vi "set C1 trigger.vi"(8 "error in (no error)":errorcluster, 10 "free run?":bool, 11 "Waveform in":refnum<class "Waveform.lvclass">) -> (0 "error out":errorcluster, 3 "Waveform out":refnum<class "Waveform.lvclass">)   [LabVIEW 2012, in "Waveform.lvclass"]
uses:
  Waveform.lvclass
  Waveform.lvclass/Waveform.ctl
  <vilib>/DAQmx/configure/trigger.llb/DAQmx Start Trigger (Digital Edge).vi
  <vilib>/DAQmx/configure/trigger.llb/DAQmx Start Trigger (None).vi
  <resource>/objmgr/daqmx.rc
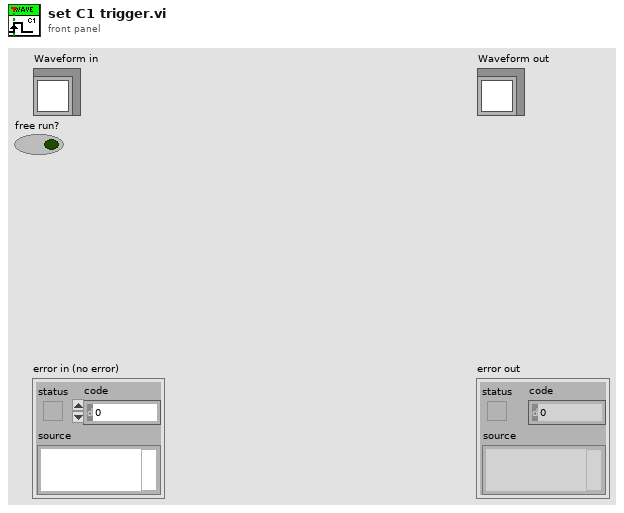
[diagram p1: front panel]
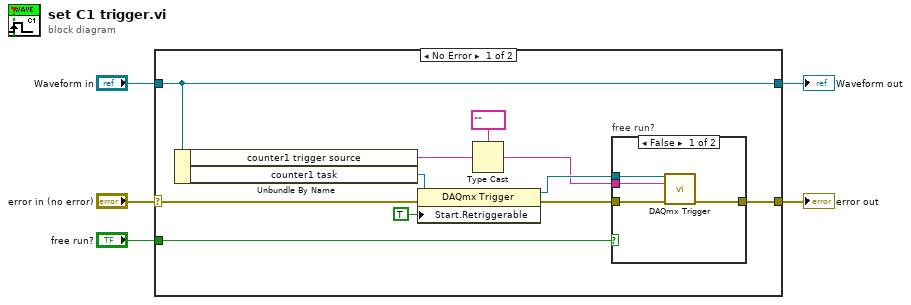
[diagram p0: block diagram]
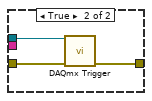
[diagram p2: hidden frame]
diagram:
  n1 = case shown="No Error" "error in (no error)" {
    selector: "error in (no error)" -> [w12 w25]
    tunnel: [w11 w25] -> w4
    tunnel: [w16 w24] -> w2
    tunnel: "Waveform in" -> [w16 w24]
    tunnel: "free run?" -> [w6 _]
    frame No Error {
      n2 = Unbundle By Name(w16) -> ("counter1 trigger source"=w9:string, "counter1 task"=w15:refnum<k21>)
      n3 = property class="DAQmx Trigger"(reference=w15, error in=w12, "Start.Retriggerable"=TRUE) -> (reference out=w10:refnum<k21>, error out=w13:errorcluster)
      n4 = Type Cast(type=tag "" ("source"), x=w9) -> (*(type *) &x=w8:tag)
      n5 = case "free run?" shown="False" w6 {
        tunnel: w13 -> [w20 w23]
        tunnel: [w19 w22] -> w11
        tunnel: w10 -> [w18 w21]
        tunnel: w8 -> [w17 _]
        frame False {
          n6 = call-poly <vilib>:"DAQmx Trigger.vi"("task/channels in"=w18, "source"=w17, "error in"=w20) -> ("error out"=w19:errorcluster)  [unwired: 11 in, 1 out]
        }
        frame True {
          n7 = call-poly <vilib>:"DAQmx Trigger.vi"("task/channels in"=w21, "error in"=w23) -> ("error out"=w22:errorcluster)  [unwired: 12 in, 1 out]
        }
      }
    }
    frame Error {
    }
  }
  "error out" <- w4
  "Waveform out" <- w2
